vi "TCP_WRITE_READ_SV.vi"(8 "error in (no error)":errorcluster, 10 "command":string, 11 "TCP Network Connection in":refnum<k5>) -> (0 "error out":errorcluster, 3 "TCP Network Connection out":refnum<k5>)   [LabVIEW 2016]
uses:
  TCP_GV.vi
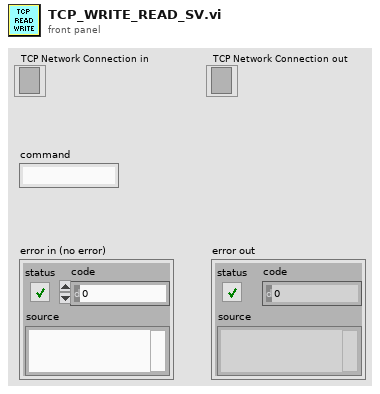
[diagram p1: front panel]
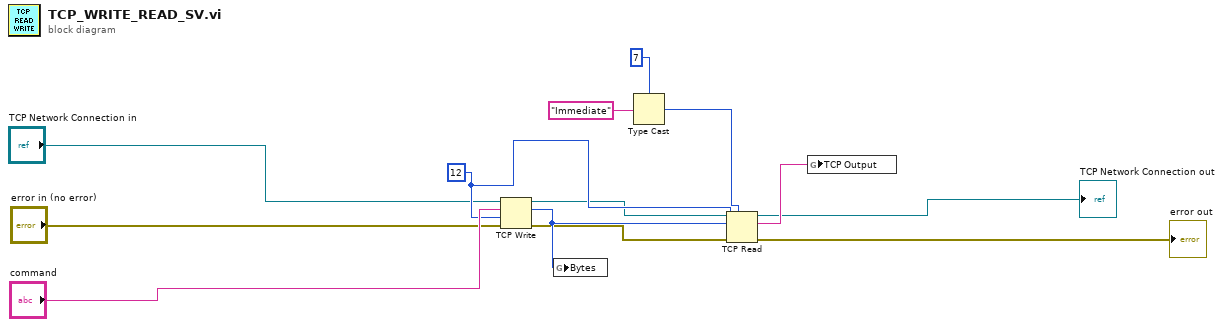
[diagram p0: block diagram]
diagram:
  w10 = 12 ("timeout ms (25000)")
  n1 = TCP Write(connection ID="TCP Network Connection in", data in="command", error in (no error)="error in (no error)", 9:w10) -> (connection ID out=w3:refnum<k5>, bytes written=w12:i32, error out=w4:errorcluster)
  n2 = global write "TCP_GV.vi" "Bytes"(w12) -> ()
  n3 = Type Cast(type=7, x="Immediate") -> (*(type *) &x=w9:i32)
  n4 = TCP Read(connection ID=w3, bytes to read=w12, error in (no error)=w4, 7:w9, 9:w10) -> (connection ID out=→"TCP Network Connection out":refnum<k5>, data out=w13:string, error out=→"error out":errorcluster)
  n5 = global write "TCP_GV.vi" "TCP Output"(w13) -> ()
